vi "AttributesDataStorage.vi"() -> ()   [LabVIEW 2014, in "examples.lvlib"]
uses:
  vis/tango_vi.llb/_TangoState_t.ctl
  examples.lvlib
  vis/tango_vi.llb/tango.lvlib
panel:
  in  "enum":T1(ring)
  in  "stri":string[][](array[string])
  in  "strsp":string[](array[string])
  in  "str":string
  out "booli":bool[][](array[boolean])
  out "boolsp":bool[](array[boolean])
  in  "statei":T2[][](array[typedef])
  in  "statesp":T2[](array[typedef])
  in  "state":T2=enum."UNKNOWN"
  out "bool":bool
  out "u8":u8
  out "i16":i16
  out "u16":u16
  out "i32":i32
  out "u32":u32
  out "i64":i64
  out "u64":u64
  out "sgl":sgl
  out "dbl":dbl
  out "u8sp":u8[](array[numeric])
  out "i16sp":i16[](array[numeric])
  out "u16sp":u16[](array[numeric])
  out "u32sp":u32[](array[numeric])
  out "i32sp":i32[](array[numeric])
  out "i64sp":i64[](array[numeric])
  out "dblsp":dbl[](array[numeric])
  out "sglsp":sgl[](array[numeric])
  out "u64sp":u64[](array[numeric])
  out "u8i":u8[][](array[numeric])
  out "i16i":i16[][](array[numeric])
  out "u16i":u16[][](array[numeric])
  out "u32i":u32[][](array[numeric])
  out "i64i":i64[][](array[numeric])
  out "u64i":u64[][](array[numeric])
  out "sgli":sgl[][](array[numeric])
  out "i32i":i32[][](array[numeric])
  out "dbli":dbl[][](array[numeric])
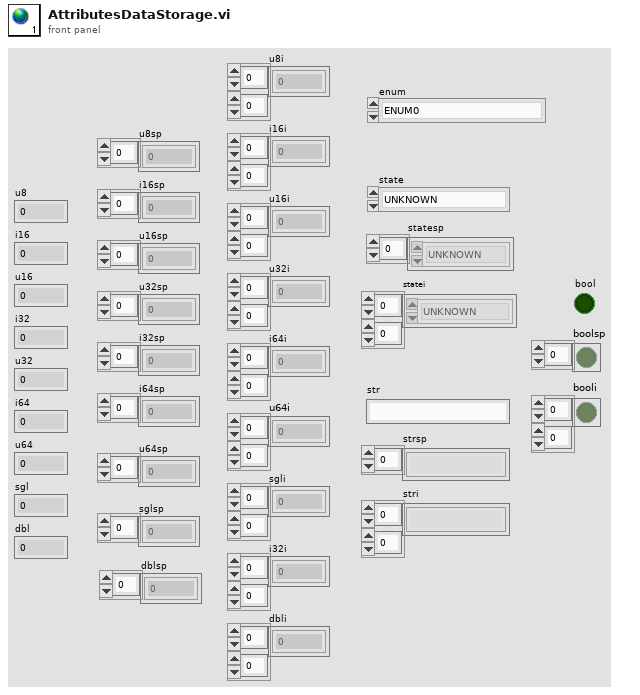
[diagram p1: front panel]
types:
  T1 = enum16{"ENUM0", "ENUM1", "ENUM2", "ENUM3", "UNKNOWN"}
  T2 = typedef "tango.lvlib/_TangoState_t.ctl" = enum32{"ON", "OFF", "CLOSE", "OPEN", "INSERT", "EXTRACT", "MOVING", "STANDBY", "FAULT", "INIT", "RUNNING", "ALARM", "DISABLE", "UNKNOWN"}
diagram:
